vi "crit5.vi"(5 "ArrayIn":dbl[](array[numeric])) -> (0 "lin":dbl[](array[numeric]), 1 "max value":dbl, 3 "C":dbl[](array[numeric]) format="%#_3g")   [LabVIEW 2010]
uses:
  <vilib>/Analysis/baseanly.llb/A x Vector.vi
  <vilib>/Analysis/baseanly.llb/Vector x A.vi
  <vilib>/Analysis/NI_AALBase.lvlib
panel:
  # "перегиб (пока нет)"
  # "выпуклость"
  # "наклон"
  # "среднее"
  # "если наклон резко изменился - скачок\nесли выпуклость больше наклона - линейная аппроксимация не годится"
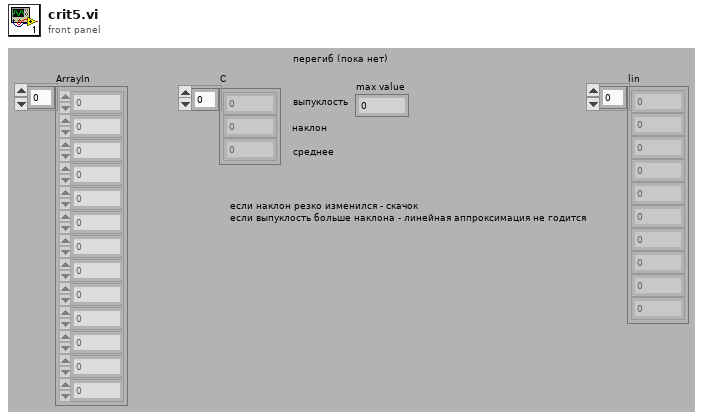
[diagram p1: front panel]
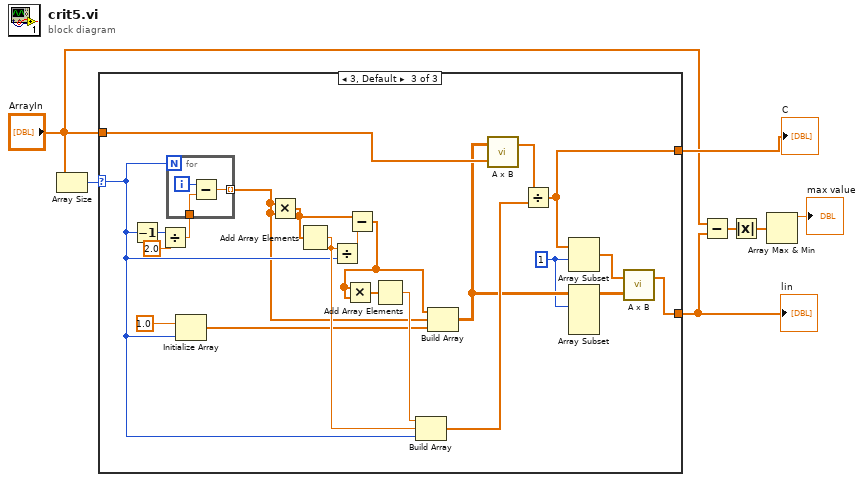
[diagram p0: block diagram]
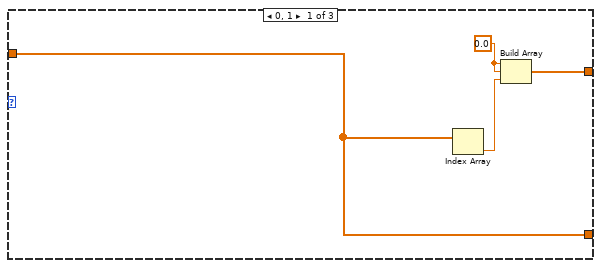
[diagram p2: hidden frame]
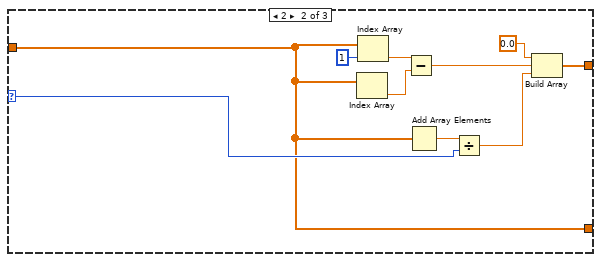
[diagram p3: hidden frame]
diagram:
  n1 = Array Size(array="ArrayIn") -> (size(s)=w7:i32)
  n2 = case shown="3, Default" w7 {
    selector: w7 -> [_ w20 w34]
    tunnel: "ArrayIn" -> [w10 w14 w41]
    tunnel: [w10 w14 w27] -> w4
    tunnel: [w11 w18 w26] -> w6
    frame 0, 1 {
      w8 = 0.0 ("element")
      n3 = Index Array(array=w10) -> (element=w9:dbl)  [unwired: 1 in]
      n4 = Build Array(w8, w8, w9) -> (w11:dbl[])
    }
    frame 2 {
      n5 = Index Array(array=w14) -> (element=w15:dbl)  [unwired: 1 in]
      n6 = Index Array(array=w14, index=1) -> (element=w16:dbl)
      n7 = Subtract(x=w16, y=w15) -> (x-y=w13:dbl)
      n8 = Add Array Elements(numeric array=w14) -> (sum=w21:dbl)
      n9 = Divide(x=w21, y=w20) -> (x/y=w19:dbl)
      n10 = Build Array(0.0 ("element"), w13, w19) -> (w18:dbl[])
    }
    frame 3, Default {
      w22 = 1 ("index")
      n11 = Decrement(x=w34) -> (x-1=w37:i32)
      n12 = Divide(x=w37, y=2.0) -> (x/y=w38:dbl)
      n13 = for {
        N: w34 -> [_]
        tunnel: w38 -> [w45]
        tunnel: [w44] -> w30 mode=indexing
        i -> [w46]
        n14 = Subtract(x=w46, y=w45) -> (x-y=w44:dbl)
      }
      n15 = Initialize Array(1.0 ("element"), w34) -> (w29:dbl[])
      n16 = Multiply(x=w30, y=w30) -> (x*y=w33:dbl[])
      n17 = Add Array Elements(numeric array=w33) -> (sum=w43:dbl)
      n18 = Divide(x=w43, y=w34) -> (x/y=w36:dbl)
      n19 = Subtract(x=w33, y=w36) -> (x-y=w31:dbl[])
      n20 = Multiply(x=w31, y=w31) -> (x*y=w40:dbl[])
      n21 = Add Array Elements(numeric array=w40) -> (sum=w42:dbl)
      n22 = Build Array(w42, w43, w34) -> (w28:dbl[])
      n23 = Build Array(w31, w30, w29) -> (w25:dbl[][])
      n24 = call-poly <vilib>:"A x B.vi"("Vector"=w41, "A"=w25) -> ("A x Vector"=w32:dbl[])  [unwired: 1 out]
      n25 = Divide(x=w32, y=w28) -> (x/y=w26:dbl[])
      n26 = Array Subset(array=w26, index=w22) -> (w23:dbl[])  [unwired: 1 in]
      n27 = Array Subset(array=w25, index (row)=w22) -> (w24:dbl[][])  [unwired: 3 in]
      n28 = call-poly <vilib>:"A x B.vi"("Matrix A"=w24, "Vector V'"=w23) -> ("V' x A"=w27:dbl[])  [unwired: 1 out]
    }
  }
  "C" <- w6
  "lin" <- w4
  n29 = Subtract(x="ArrayIn", y=w4) -> (x-y=w3:dbl[])
  n30 = Absolute Value(x=w3) -> (abs(x)=w2:dbl[])
  n31 = Array Max & Min(array=w2) -> (max value=→"max value":dbl)  [unwired: 3 out]
